vi "Test Host VI.vi"() -> ()   [LabVIEW 2026]
uses:
  <vilib>/rvi/DesktopExecutionNode/Execution/niFpgaDEN_Execute.vi
  <vilib>/rvi/DesktopExecutionNode/DesktopExecutionNode.xnode
panel:
  out "Mod8/DO7":bool
  out "Mod8/DO6":bool
  out "Mod8/DO5":bool
  out "Mod8/DO4":bool
  out "Mod8/DO3":bool
  out "Mod8/DO2":bool
  out "Mod8/DO1":bool
  out "Mod8/DO0":bool
  in  "Mod8/DI7":bool
  in  "Mod8/DI6":bool
  in  "Mod8/DI5":bool
  in  "Mod8/DI4":bool
  in  "Mod8/DI3":bool
  in  "Mod8/DI2":bool
  in  "Mod8/DI1":bool
  in  "Mod8/DI0":bool
  out "Time Left (ms)":i32
  out "Score":i16
  in  "Boolean array 4":bool[](array[boolean])=[FALSE, FALSE, FALSE, FALSE, FALSE, FALSE, FALSE, FALSE, FALSE, FALSE, FALSE, FALSE, FALSE, FALSE, FALSE, FALSE]
  in  "Boolean array 3":bool[](array[boolean])=[FALSE, FALSE, FALSE, FALSE, FALSE, FALSE, FALSE, FALSE, FALSE, FALSE, FALSE, FALSE, FALSE, FALSE, FALSE, FALSE]
  out "Boolean array 2":bool[](array[boolean])
  out "Boolean array":bool[](array[boolean])
  out "Iteration":i32
  in  "stop":bool
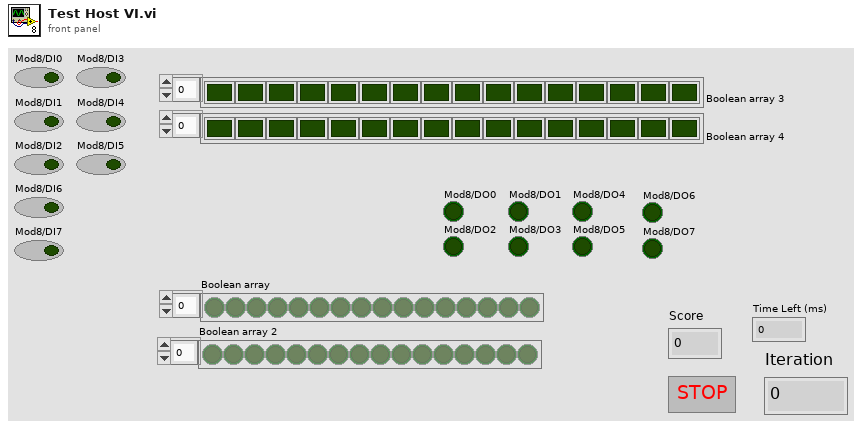
[diagram p1: front panel]
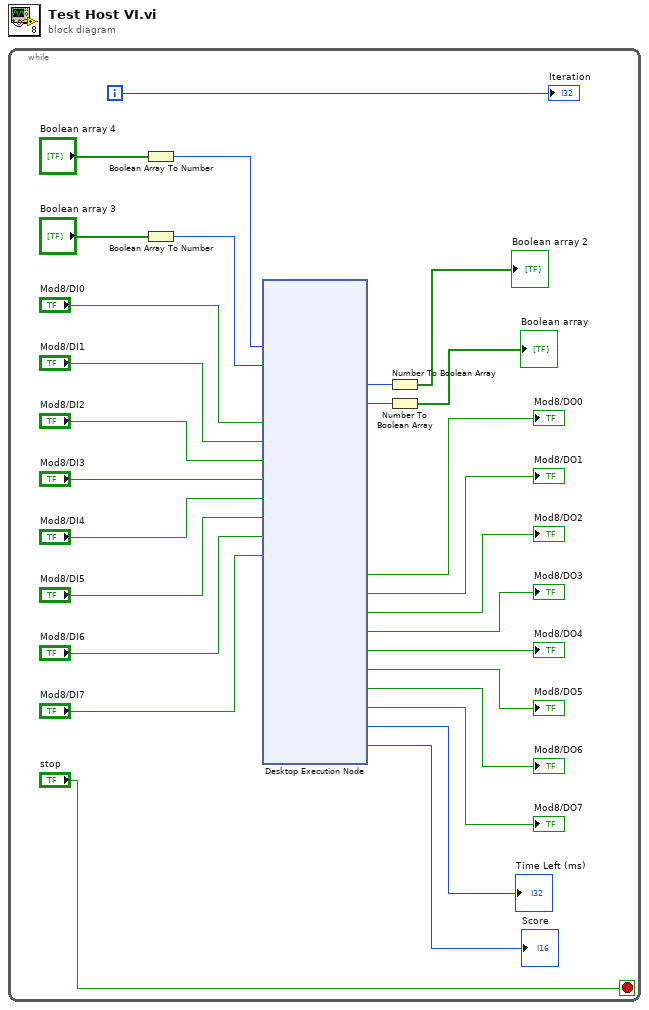
[diagram p0: block diagram]
diagram:
  n1 = while {
    i -> [w27]
    stop <- "stop" stop-if-true
    n2 = Boolean Array To Number(Boolean array="Boolean array 4") -> (number=w17:u32)
    n3 = Boolean Array To Number(Boolean array="Boolean array 3") -> (number=w22:u32)
    n4 = xnode "Desktop Execution Node"("Mod5/DI15:0"=w17, "Mod7/DI15:0"=w22, "Mod8/DI0"="Mod8/DI0", "Mod8/DI1"="Mod8/DI1", "Mod8/DI2"="Mod8/DI2", "Mod8/DI3"="Mod8/DI3", "Mod8/DI4"="Mod8/DI4", "Mod8/DI5"="Mod8/DI5", "Mod8/DI6"="Mod8/DI6", "Mod8/DI7"="Mod8/DI7") -> ("Mod5/DO15:0"=w24:u16, "Mod7/DO15:0"=w26:u16, "Mod8/DO0"=→"Mod8/DO0":bool, "Mod8/DO1"=→"Mod8/DO1":bool, "Mod8/DO2"=→"Mod8/DO2":bool, "Mod8/DO3"=→"Mod8/DO3":bool, "Mod8/DO4"=→"Mod8/DO4":bool, "Mod8/DO5"=→"Mod8/DO5":bool, "Mod8/DO6"=→"Mod8/DO6":bool, "Mod8/DO7"=→"Mod8/DO7":bool, "Time Left (ms)"=→"Time Left (ms)":i32, "Score"=→"Score":u16)  [unwired: 1 in, 1 out]
    n5 = Number To Boolean Array(number=w24) -> (Boolean array=→"Boolean array 2":bool[])
    n6 = Number To Boolean Array(number=w26) -> (Boolean array=→"Boolean array":bool[])
    "Iteration" <- w27
  }
